vi "write_command.vi"(8 "error in (no error)":errorcluster, 10 "command (without terminating \"\\n\")":string, 11 "DL090602SutterMP285Stage in":refnum<class "StageMMS2015ASI.lvclass">) -> (0 "error out":errorcluster, 3 "DL090602SutterMP285Stage out":refnum<class "StageMMS2015ASI.lvclass">)   [LabVIEW 2010, in "StageMMS2015ASI.lvclass"]
uses:
  StageMMS2015ASI.lvclass
  StageMMS2015ASI.lvclass/StageMMS2015ASI.ctl
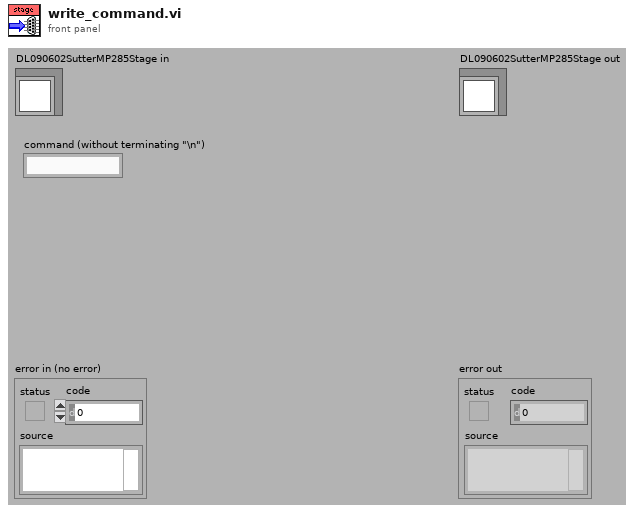
[diagram p1: front panel]
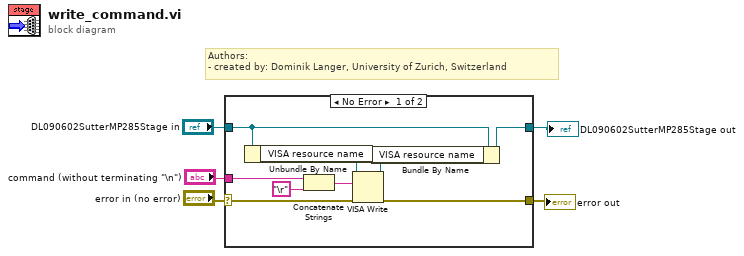
[diagram p0: block diagram]
diagram:
  # "Authors: \n- created by: Dominik Langer, University of Zurich, Switzerland"
  n1 = case shown="No Error" "error in (no error)" {
    selector: "error in (no error)" -> [w13 w16]
    tunnel: [w12 w16] -> w4
    tunnel: [w9 w15] -> w2
    tunnel: "DL090602SutterMP285Stage in" -> [w10 w15]
    tunnel: "command (without terminating \"\\n\")" -> [w8 _]
    frame No Error {
      n2 = Unbundle By Name(w10) -> ("VISA resource name"=w7:refnum<visa-resource-name>)
      n3 = Concatenate Strings(w8, "\r") -> (w6:string)
      n4 = VISA Write(VISA resource name=w7, write buffer=w6, error in (no error)=w13) -> (VISA resource name out=w11:refnum<visa-resource-name>, error out=w12:errorcluster)  [unwired: 1 out]
      n5 = Bundle By Name(cluster=w10, "VISA resource name"=w11) -> (w9:refnum<class "StageMMS2015ASI.lvclass">)
    }
    frame Error {
    }
  }
  "error out" <- w4
  "DL090602SutterMP285Stage out" <- w2
